vi "Update controls.vi"(8 "error in (no error)":errorcluster caption="entrée d'erreur (pas d'erreur)", 10 "IHM Data refnum":T1, 11 "Front Panel status":T2) -> (0 "error out":errorcluster caption="sortie d'erreur")   [LabVIEW 2013, in "IHM Control.lvlib"]
doc: "Le VI Update Controls, permet la modification de l'affichage des bouton de la face avant du programme Main."
uses:
  IHM Control.lvlib
  Front Panel Status.ctl
  MHL UI Ref.ctl
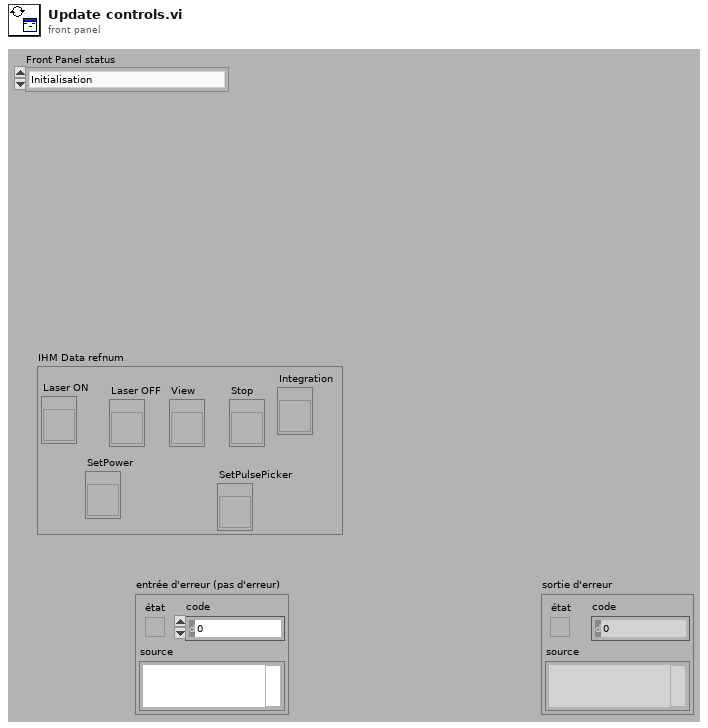
[diagram p1: front panel]
types:
  T1 = typedef "IHM Control.lvlib/MHL UI Ref.ctl" = cluster{"View":refnum<vi>, "Stop":refnum<vi>, "Laser OFF":refnum<vi>, "Laser ON":refnum<vi>, "Integration":refnum<vi>, "SetPower":refnum<vi>, "SetPulsePicker":refnum<vi>}
  T2 = typedef "IHM Control.lvlib/Front Panel Status.ctl" = enum16{"Initialisation", "Enable Laser", "Enable Camera", "Disable Laser", "Disable Camera"}
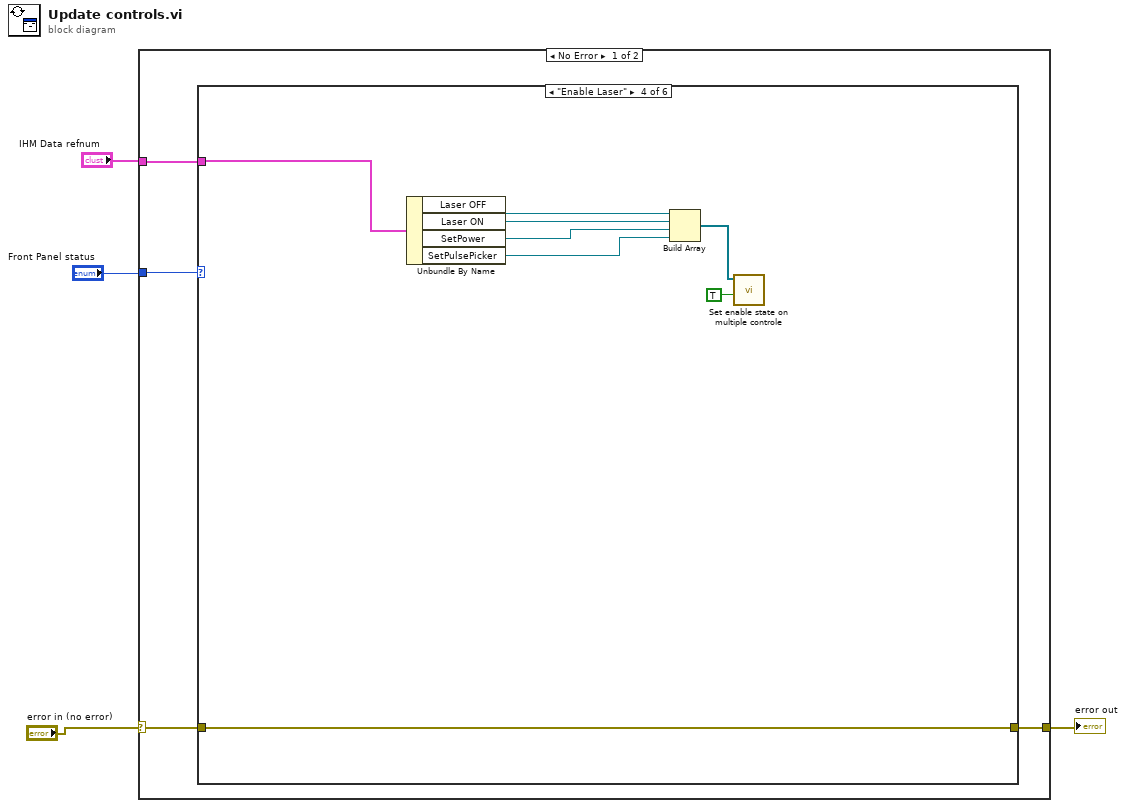
[diagram p0: block diagram]
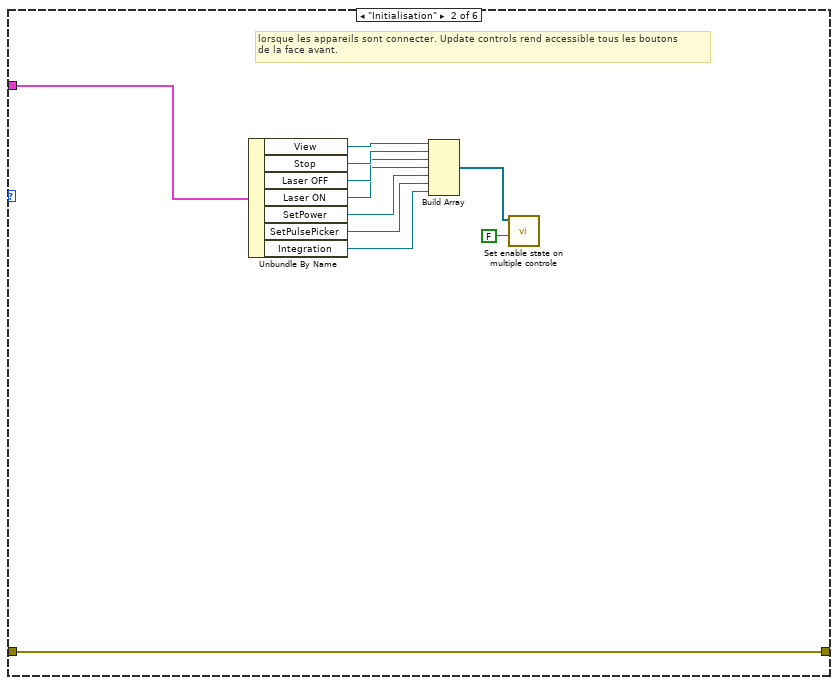
[diagram p3: hidden frame]
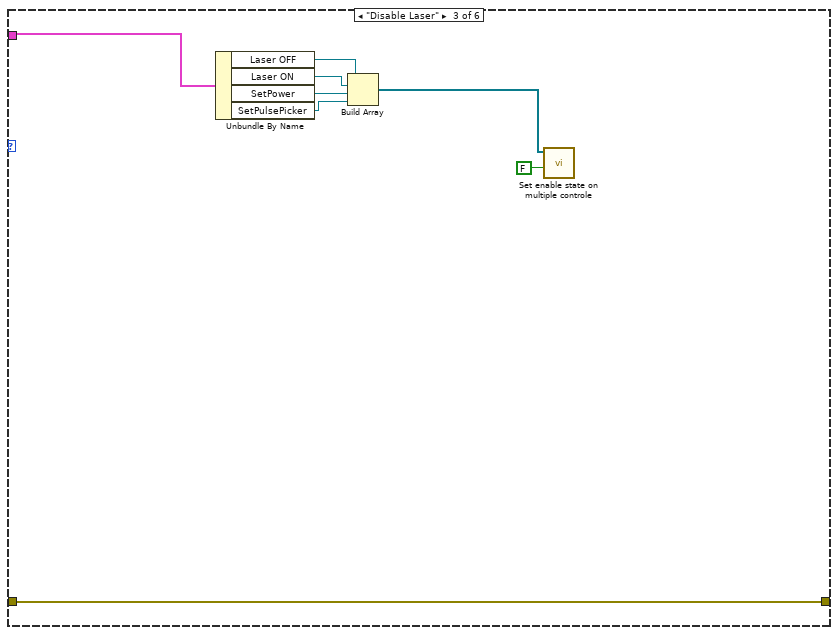
[diagram p4: hidden frame]
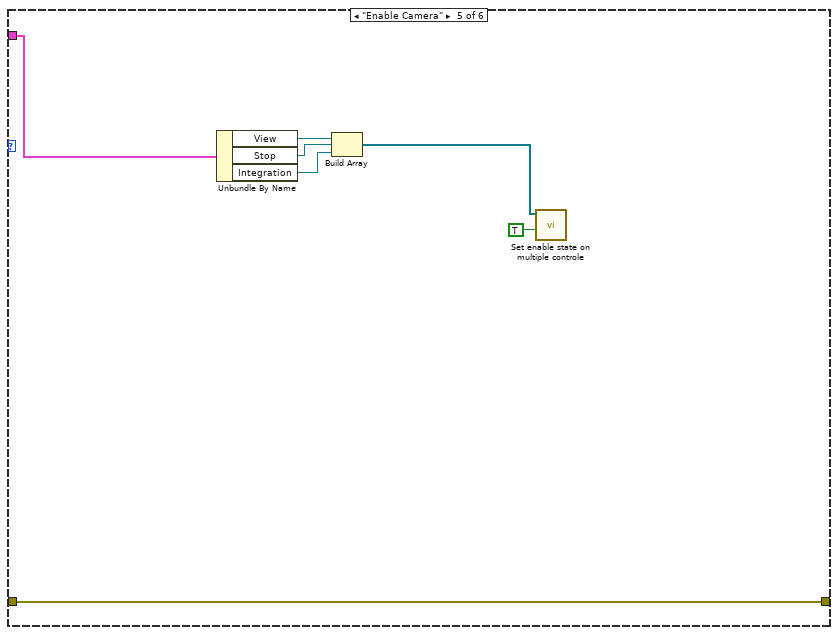
[diagram p5: hidden frame]
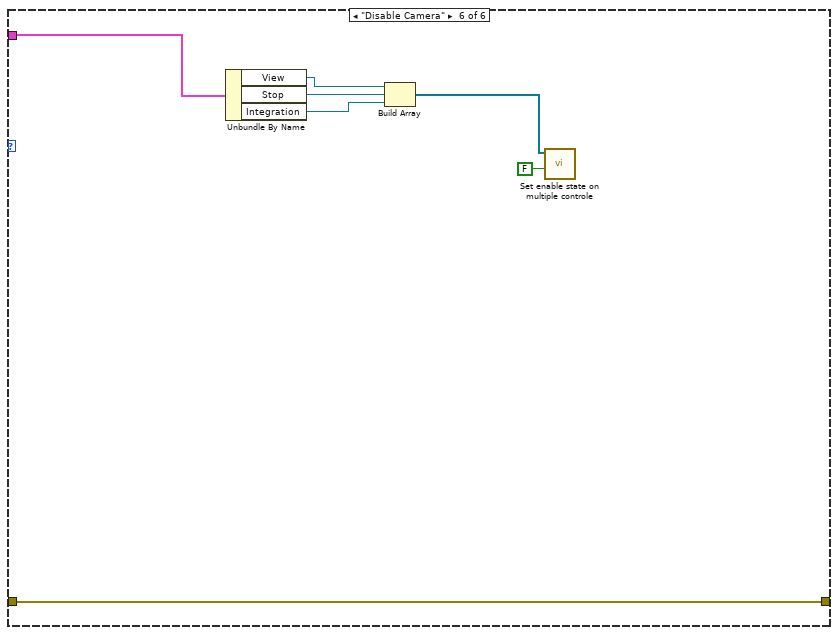
[diagram p6: hidden frame]
diagram:
  n1 = case shown="No Error" "error in (no error)" {
    selector: "error in (no error)" -> [w6 w51]
    tunnel: "Front Panel status" -> [w8 _]
    tunnel: "IHM Data refnum" -> [w7 _]
    tunnel: [w5 w51] -> w2
    frame No Error {
      n2 = case shown="\"Enable Laser\"" w8 {
        tunnel: w7 -> [_ w20 w26 w31 w39 w48]
        tunnel: [w9 w19 w28 w36 w43 w50] -> w5
        tunnel: w6 -> [w9 w19 w28 w36 w43 w50]
        frame Default {
        }
        frame "Initialisation" {
          # "lorsque les appareils sont connecter. Update controls rend accessible tous les boutons\nde la face avant."
          n3 = Unbundle By Name(w20) -> ("View"=w17:refnum<vi>, "Stop"=w16:refnum<vi>, "Laser OFF"=w15:refnum<vi>, "Laser ON"=w14:refnum<vi>, "SetPower"=w13:refnum<vi>, "SetPulsePicker"=w12:refnum<vi>, "Integration"=w11:refnum<vi>)
          n4 = Build Array(w17, w16, w15, w14, w13, w12, w11) -> (w10:refnum<vi>[])
          n5 = call "Set enable state on multiple controle.vi"("Booléen"=FALSE, "Ref. Tab"=w10) -> ()  [unwired: 10 in]
        }
        frame "Disable Laser" {
          n6 = Unbundle By Name(w26) -> ("Laser OFF"=w22:refnum<vi>, "Laser ON"=w23:refnum<vi>, "SetPower"=w25:refnum<vi>, "SetPulsePicker"=w21:refnum<vi>)
          n7 = Build Array(w22, w23, w25, w21) -> (w24:refnum<vi>[])
          n8 = call "Set enable state on multiple controle.vi"("Booléen"=FALSE, "Ref. Tab"=w24) -> ()  [unwired: 10 in]
        }
        frame "Enable Laser" {
          n9 = Unbundle By Name(w31) -> ("Laser OFF"=w30:refnum<vi>, "Laser ON"=w34:refnum<vi>, "SetPower"=w33:refnum<vi>, "SetPulsePicker"=w29:refnum<vi>)
          n10 = Build Array(w30, w34, w33, w29) -> (w32:refnum<vi>[])
          n11 = call "Set enable state on multiple controle.vi"("Booléen"=TRUE, "Ref. Tab"=w32) -> ()  [unwired: 10 in]
        }
        frame "Enable Camera" {
          n12 = Unbundle By Name(w39) -> ("View"=w41:refnum<vi>, "Stop"=w38:refnum<vi>, "Integration"=w37:refnum<vi>)
          n13 = Build Array(w41, w38, w37) -> (w42:refnum<vi>[])
          n14 = call "Set enable state on multiple controle.vi"("Booléen"=TRUE, "Ref. Tab"=w42) -> ()  [unwired: 10 in]
        }
        frame "Disable Camera" {
          n15 = Unbundle By Name(w48) -> ("View"=w47:refnum<vi>, "Stop"=w46:refnum<vi>, "Integration"=w45:refnum<vi>)
          n16 = Build Array(w47, w46, w45) -> (w44:refnum<vi>[])
          n17 = call "Set enable state on multiple controle.vi"("Booléen"=FALSE, "Ref. Tab"=w44) -> ()  [unwired: 10 in]
        }
      }
    }
    frame Error {
    }
  }
  "error out" <- w2
